vi "saveDataMN.vi"(8 "error in (no error)":errorcluster, 10 "data":T1[](array[typedef]), 11 "shot":string) -> (0 "error out":errorcluster)   [LabVIEW 2017]
uses:
  models/dataForSave.ctl
  <vilib>/MDSplus/Library/MDSplus.lvlib
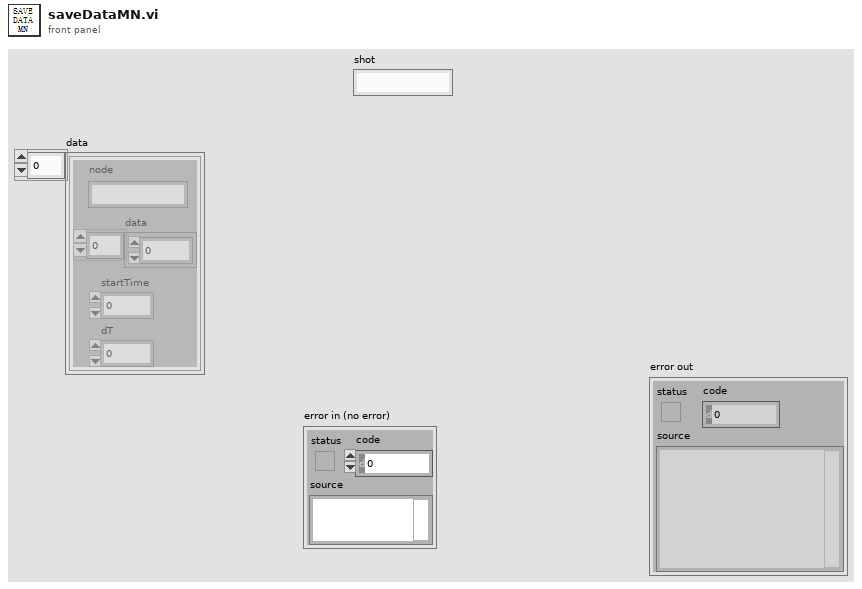
[diagram p1: front panel]
types:
  T1 = typedef "dataForSave.ctl" = cluster{"node":string, "data":dbl[], "startTime":dbl, "dT":dbl}
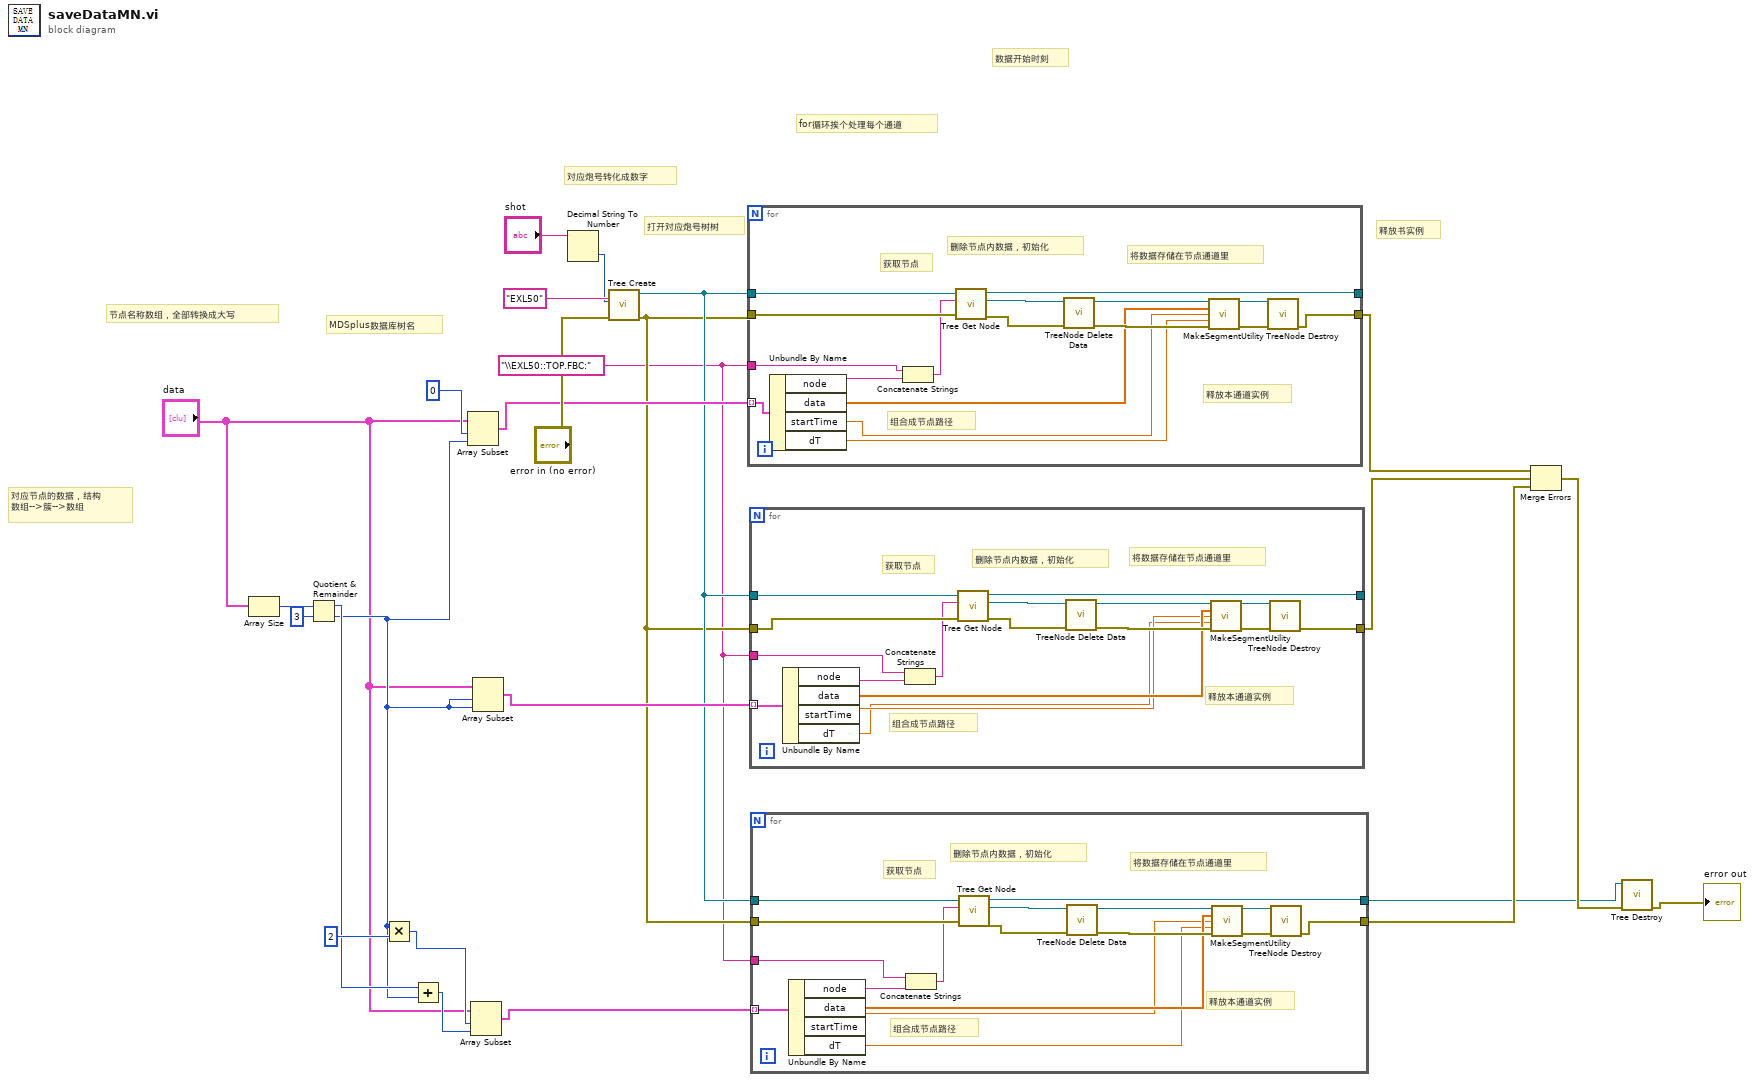
[diagram p0: block diagram]
diagram:
  w1 = "\\EXL50::TOP.FBC:" ("字符串")
  # "数据开始时刻"
  # "for循环挨个处理每个通道"
  # "释放书实例"
  # "打开对应炮号树树"
  # "对应节点的数据，结构\n数组-->簇-->数组"
  # "节点名称数组，全部转换成大写"
  # "MDSplus数据库树名"
  # "对应炮号转化成数字"
  n1 = Array Size(array="data") -> (size(s)=w21:i32)
  n2 = Quotient & Remainder(x=w21, y=3) -> (x-y*floor(x/y)=w16:i32, floor(x/y)=w5:i32)
  n3 = Multiply(x=w5, y=2) -> (x*y=w4:i32)
  n4 = Add(x=w16, y=w5) -> (x+y=w3:i32)
  n5 = Array Subset(array="data", index=0 ("索引"), length=w5) -> (w19:T1[])
  n6 = Array Subset(array="data", index=w4, length=w3) -> (w7:T1[])
  n7 = Array Subset(array="data", index=w5, length=w5) -> (w18:T1[])
  n8 = Decimal String To Number(string="shot") -> (number=w22:i32)  [unwired: 2 in, 1 out]
  n9 = call <vilib>:"Tree Create.vi"("error in (no error)"="error in (no error)", "Shot"=w22, "Name"="EXL50" ("TreeName")) -> ("error out"=w8:errorcluster, "Tree DVR out"=w9:refnum<data-value>)  [unwired: 7 in]
  n10 = for {
    tunnel: w19 -> [w31] mode=indexing
    tunnel: w8 -> [w39]
    tunnel: [w37] -> w14
    tunnel: w9 -> [w38]
    tunnel: [w36] -> _
    tunnel: w1 -> [w26]
    # "释放本通道实例"
    # "将数据存储在节点通道里"
    # "删除节点内数据，初始化"
    # "获取节点"
    # "组合成节点路径"
    n11 = Unbundle By Name(w31) -> ("node"=w29:string, "data"=w30:dbl[], "startTime"=w28:dbl, "dT"=w27:dbl)
    n12 = Concatenate Strings(w26, w29) -> (w35:string)
    n13 = call <vilib>:"Tree Get Node.vi"("error in (no error)"=w39, "Path"=w35, "Tree DVR in"=w38) -> ("error out"=w41:errorcluster, "Node out"=w40:refnum<data-value>, "Tree DVR out"=w36:refnum<data-value>)  [unwired: 6 in]
    n14 = call <vilib>:"TreeNode Delete Data.vi"("error in (no error)"=w41, "TreeNode DVR in"=w40) -> ("error out"=w34:errorcluster, "TreeNode DVR out"=w42:refnum<data-value>)  [unwired: 8 in]
    n15 = call <vilib>:"MakeSegmentUtility.vi"("TreeNode DVR in"=w42, "DBL Array"=w30, "Start time"=w28, "dt"=w27, "error in (no error)"=w34) -> ("TreeNode DVRout"=w33:refnum<data-value>, "error out"=w32:errorcluster)  [unwired: 9 in]
    n16 = call <vilib>:"TreeNode Destroy.vi"("error in (no error)"=w32, "TreeNode DVR in"=w33) -> ("error out"=w37:errorcluster)  [unwired: 9 in]
  }
  n17 = for {
    tunnel: w18 -> [w48] mode=indexing
    tunnel: w8 -> [w56]
    tunnel: [w54] -> w15
    tunnel: w9 -> [w55]
    tunnel: [w53] -> _
    tunnel: w1 -> [w43]
    # "释放本通道实例"
    # "将数据存储在节点通道里"
    # "删除节点内数据，初始化"
    # "获取节点"
    # "组合成节点路径"
    n18 = Unbundle By Name(w48) -> ("node"=w47:string, "data"=w46:dbl[], "startTime"=w45:dbl, "dT"=w44:dbl)
    n19 = Concatenate Strings(w43, w47) -> (w52:string)
    n20 = call <vilib>:"Tree Get Node.vi"("error in (no error)"=w56, "Path"=w52, "Tree DVR in"=w55) -> ("error out"=w58:errorcluster, "Node out"=w57:refnum<data-value>, "Tree DVR out"=w53:refnum<data-value>)  [unwired: 6 in]
    n21 = call <vilib>:"TreeNode Delete Data.vi"("error in (no error)"=w58, "TreeNode DVR in"=w57) -> ("error out"=w51:errorcluster, "TreeNode DVR out"=w59:refnum<data-value>)  [unwired: 8 in]
    n22 = call <vilib>:"MakeSegmentUtility.vi"("TreeNode DVR in"=w59, "DBL Array"=w46, "Start time"=w45, "dt"=w44, "error in (no error)"=w51) -> ("TreeNode DVRout"=w50:refnum<data-value>, "error out"=w49:errorcluster)  [unwired: 9 in]
    n23 = call <vilib>:"TreeNode Destroy.vi"("error in (no error)"=w49, "TreeNode DVR in"=w50) -> ("error out"=w54:errorcluster)  [unwired: 9 in]
  }
  n24 = for {
    tunnel: w7 -> [w65] mode=indexing
    tunnel: w8 -> [w73]
    tunnel: [w66] -> w13
    tunnel: w9 -> [w72]
    tunnel: [w71] -> w11
    tunnel: w1 -> [w60]
    # "释放本通道实例"
    # "将数据存储在节点通道里"
    # "删除节点内数据，初始化"
    # "获取节点"
    # "组合成节点路径"
    n25 = Unbundle By Name(w65) -> ("node"=w64:string, "data"=w63:dbl[], "startTime"=w62:dbl, "dT"=w61:dbl)
    n26 = Concatenate Strings(w60, w64) -> (w70:string)
    n27 = call <vilib>:"Tree Get Node.vi"("error in (no error)"=w73, "Path"=w70, "Tree DVR in"=w72) -> ("error out"=w75:errorcluster, "Node out"=w74:refnum<data-value>, "Tree DVR out"=w71:refnum<data-value>)  [unwired: 6 in]
    n28 = call <vilib>:"TreeNode Delete Data.vi"("error in (no error)"=w75, "TreeNode DVR in"=w74) -> ("error out"=w69:errorcluster, "TreeNode DVR out"=w76:refnum<data-value>)  [unwired: 8 in]
    n29 = call <vilib>:"MakeSegmentUtility.vi"("TreeNode DVR in"=w76, "DBL Array"=w63, "Start time"=w62, "dt"=w61, "error in (no error)"=w69) -> ("TreeNode DVRout"=w68:refnum<data-value>, "error out"=w67:errorcluster)  [unwired: 9 in]
    n30 = call <vilib>:"TreeNode Destroy.vi"("error in (no error)"=w67, "TreeNode DVR in"=w68) -> ("error out"=w66:errorcluster)  [unwired: 9 in]
  }
  n31 = Merge Errors(w14, w15, w13) -> (w12:errorcluster)
  n32 = call <vilib>:"Tree Destroy.vi"("error in (no error)"=w12, "Tree DVR in"=w11) -> ("error out"=→"error out":errorcluster)  [unwired: 9 in]
